vi "pd-demodulation.vi"(10 "Signal":dbl[](array[numeric]), 11 "Clock":dbl[](array[numeric])) -> (1 "Demodulated signal":dynamicdata(graph), 2 "Original Signal":dynamicdata(graph))   [LabVIEW 2021]
uses:
  <vilib>/Analysis/baseanly.llb/Mean (DBL).vi
  <vilib>/Analysis/NI_AALBase.lvlib
panel:
  out "middle point pos":dbl
  in  "stop":bool
  out "mean neg":dbl format="%0.2f"
  out "array size low":i32
  out "array size high":i32
  out "mean pos":dbl format="%0.2f"
  out "low":bool
  out "high":bool
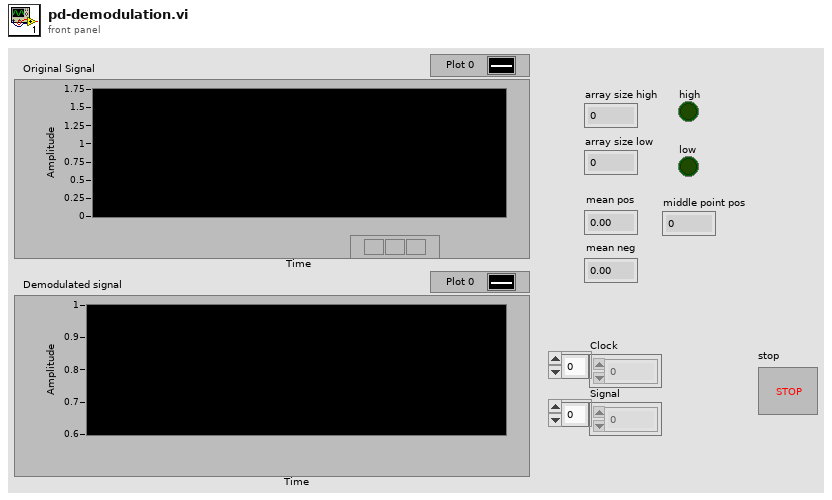
[diagram p1: front panel]
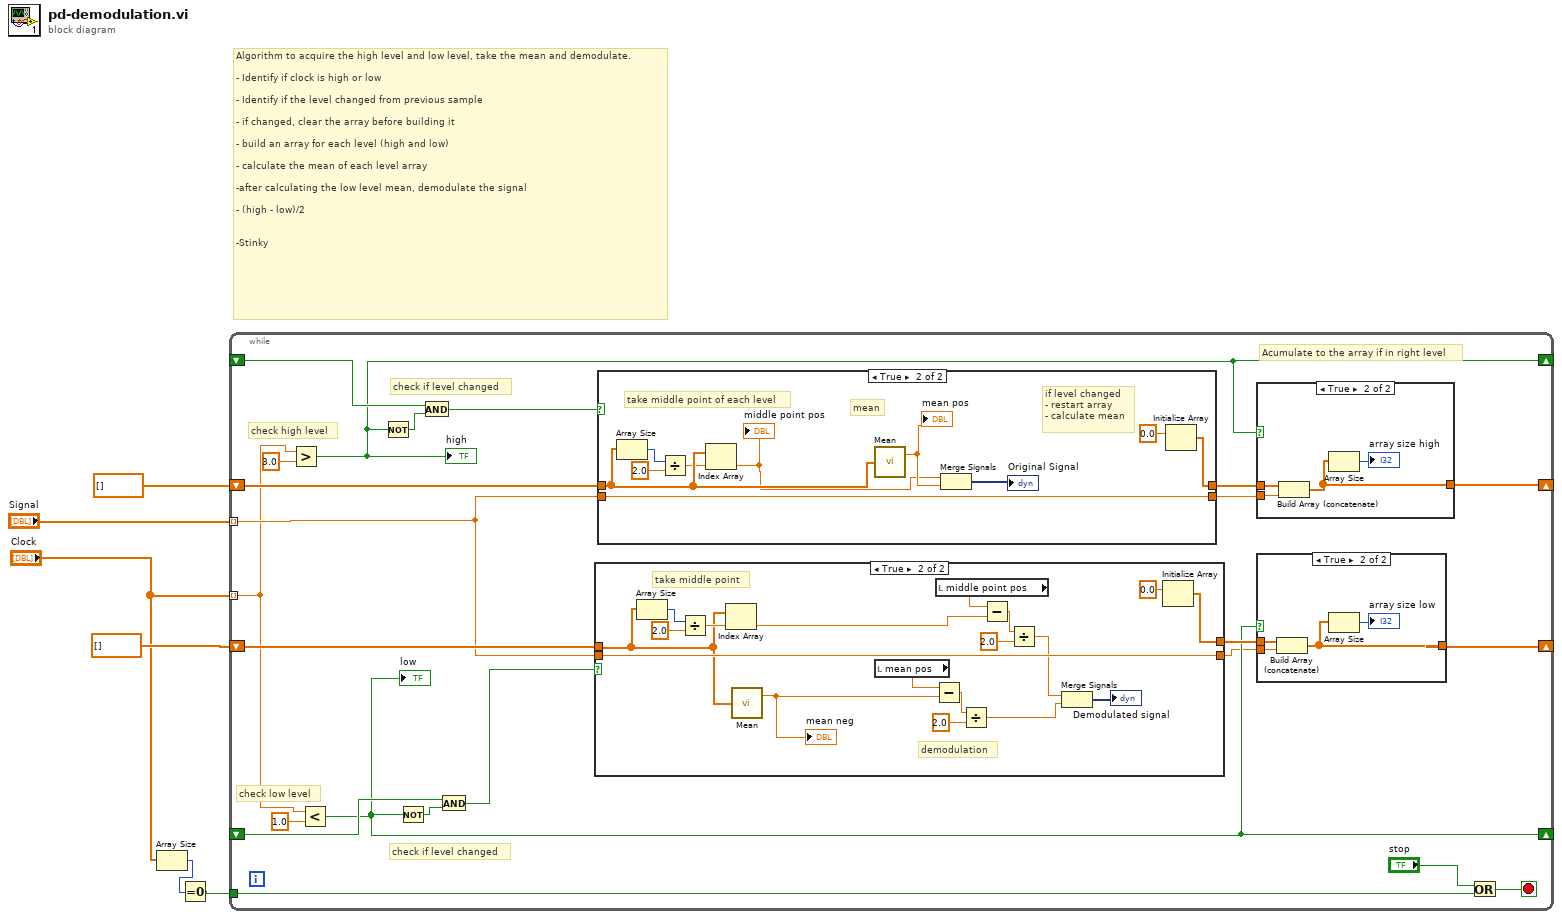
[diagram p0: block diagram]
diagram:
  # "Algorithm to acquire the high level and low level, take the mean and demodulate.\n\n- Identify if clock is high or low\n\n- Identify if the level changed from previous sample\n\n- if changed, clear the array before building it\n\n- build an array for each level (high and low)\n\n- calculate the mean of each level array\n\n-after calculating the low level mean, demodulate the signal\n\n- (high - low)/2\n\n\n-Stinky"
  n1 = Array Size(array="Clock") -> (size(s)=w3:i32)
  n2 = Equal To 0?(x=w3) -> (x = 0?=w2:bool)
  n3 = while {
    tunnel: "Clock" -> [w9] mode=indexing
    shift-right: [w26] -> _
    shift-left: dbl[] [] -> [w27]
    shift-right: [w17] -> _
    shift-left: dbl[] [] -> [w19]
    shift-right: [w16] -> _
    shift-left: _ -> [w24]
    shift-right: [w15] -> _
    shift-left: _ -> [w20]
    tunnel: "Signal" -> [w10] mode=indexing
    tunnel: w2 -> [w7]
    stop <- w12 stop-if-true
    # "Acumulate to the array if in right level"
    # "check high level"
    # "check low level"
    # "check if level changed"
    # "check if level changed"
    n4 = Greater?(x=w9, y=3.0) -> (0:w16:bool)
    "high" <- w16
    n5 = Less?(x=w9, y=1.0) -> (x < y?=w15:bool)
    "low" <- w15
    n6 = Not(x=w16) -> (.not. x?=w25:bool)
    n7 = Not(x=w15) -> (.not. x?=w21:bool)
    n8 = And(x=w24, y=w25) -> (x .and. y?=w22:bool)
    n9 = And(x=w20, y=w21) -> (x .and. y?=w14:bool)
    n10 = case shown="True" w14 {
      tunnel: [w43 w60] -> w18
      tunnel: w19 -> [w43 w52]
      tunnel: [w42 w59] -> w8
      tunnel: w10 -> [w42 w59]
      frame False {
      }
      frame True {
        # "demodulation"
        # "take middle point"
        n11 = Array Size(array=w52) -> (size(s)=w54:i32)
        n12 = Divide(x=w54, y=2.0) -> (x/y=w53:dbl)
        n13 = Index Array(array=w52, index=w53) -> (element=w51:dbl)
        n14 = call-poly <vilib>:"Mean.vi"("X"=w52) -> ("mean"=w44:dbl)  [unwired: 1 out]
        "mean neg" <- w44
        n15 = local read "mean pos"() -> (w45:dbl)
        n16 = Subtract(x=w45, y=w44) -> (x-y=w49:dbl)
        n17 = local read "middle point pos"() -> (w56:dbl)
        n18 = Divide(x=w49, y=2.0) -> (x/y=w46:dbl)
        n19 = Subtract(x=w56, y=w51) -> (x-y=w57:dbl)
        n20 = Divide(x=w57, y=2.0) -> (x/y=w47:dbl)
        n21 = Merge Signals(w47, w46) -> (→"Demodulated signal":dynamicdata)
        n22 = Initialize Array(0.0 ("element")) -> (w60:dbl[])  [unwired: 1 in]
      }
    }
    n23 = case shown="True" w22 {
      tunnel: [w31 w40] -> w23
      tunnel: w27 -> [w31 w36]
      tunnel: [w30 w39] -> w11
      tunnel: w10 -> [w30 w39]
      frame False {
      }
      frame True {
        # "mean"
        # "take middle point of each level"
        # "if level changed\n- restart array\n- calculate mean"
        n24 = Array Size(array=w36) -> (size(s)=w37:i32)
        n25 = Divide(x=w37, y=2.0) -> (x/y=w35:dbl)
        n26 = Index Array(array=w36, index=w35) -> (element=w32:dbl)
        "middle point pos" <- w32
        n27 = call-poly <vilib>:"Mean.vi"("X"=w36) -> ("mean"=w33:dbl)  [unwired: 1 out]
        "mean pos" <- w33
        n28 = Merge Signals(w32, w33) -> (→"Original Signal":dynamicdata)
        n29 = Initialize Array(0.0 ("element")) -> (w40:dbl[])  [unwired: 1 in]
      }
    }
    n30 = case shown="True" w16 {
      tunnel: w23 -> [w67 w71]
      tunnel: [w67 w70] -> w26
      tunnel: w11 -> [_ w68]
      frame False {
      }
      frame True {
        n31 = Build Array (concatenate)(w71, w68) -> (w70:dbl[])
        n32 = Array Size(array=w70) -> (size(s)=→"array size high":i32)
      }
    }
    n33 = case shown="True" w15 {
      tunnel: w18 -> [w62 w66]
      tunnel: w8 -> [_ w65]
      tunnel: [w62 w64] -> w17
      frame False {
      }
      frame True {
        n34 = Build Array (concatenate)(w66, w65) -> (w64:dbl[])
        n35 = Array Size(array=w64) -> (size(s)=→"array size low":i32)
      }
    }
    n36 = Or(x="stop", y=w7) -> (x .or. y?=w12:bool)
  }
